vi "ResonanceAnalyzer.vi"() -> ()   [LabVIEW 2015]
uses:
  <vilib>/imath/engines/lvmath2/RunTimeEngine/Managers/WorkSpace/UID Generator.vi
  <vilib>/imath/engines/lvmath2/RunTimeEngine/RunTimeType/NIMS_RunTimeType_From StrictType (excl LVString).vi
  <instcachedir>/0/NIMS_RunTimeType_From StrictType (excl LVString)_EB1C38A9BC5048DA9ABDA8F781E54D21.lvgen/NIMS_RunTimeType_From StrictType (excl LVString)_EB1C38A9BC5048DA9ABDA8F781E54D21_000.vi
  <vilib>/imath/engines/lvmath2/RunTimeEngine/LocalVariableDefStatement/MC_LocalVariableDefStatement_Display.vi
  <vilib>/imath/engines/lvmath2/RunTimeEngine/Managers/SymbolTable/Clear UID.vi
  <vilib>/imath/engines/lvmath2/RunTimeEngine/NodeEndStatement/NIMS_NodeEndStatement_Output.vi
  <instcachedir>/0/NIMS_NodeEndStatement_Output_53EC0D466D134D7ABD903AC30B43404B.lvgen/NIMS_NodeEndStatement_Output_53EC0D466D134D7ABD903AC30B43404B_001.vi
  <vilib>/imath/engines/lvmath2/RunTimeEngine/ErrorHandling/NIMS_Finalize Error.vi
  <vilib>/Utility/file.llb/Read Delimited Spreadsheet (DBL).vi
  <vilib>/imath/engines/lvmath2/RunTimeEngine/Managers/SymbolTable/NIMS_WorkSpace.lvlib
panel:
  out "Array":dbl[](array[numeric])
  out "XY Graph":cluster{"all rows":dbl[], "all rows":dbl[]}(graph)
  in  "Tab Control":enum32{"Simulation", "Experiment"}(tab)
  in  "Input Parameters":T1
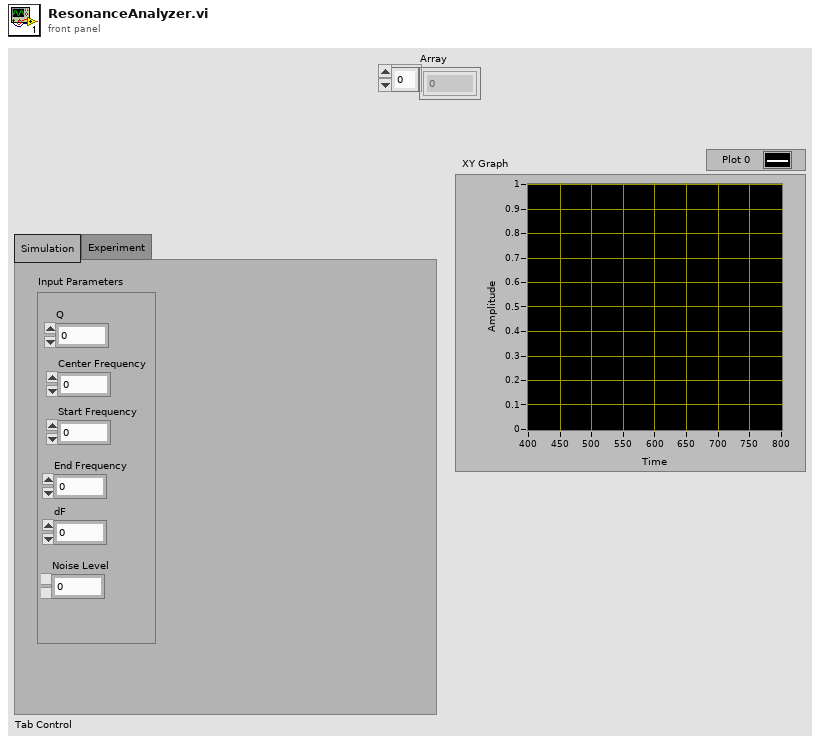
[diagram p1: front panel]
types:
  T1 = cluster{"Q":dbl, "Center Frequency":dbl, "Start Frequency":dbl, "End Frequency":dbl, "dF":dbl, "Noise Level":dbl}
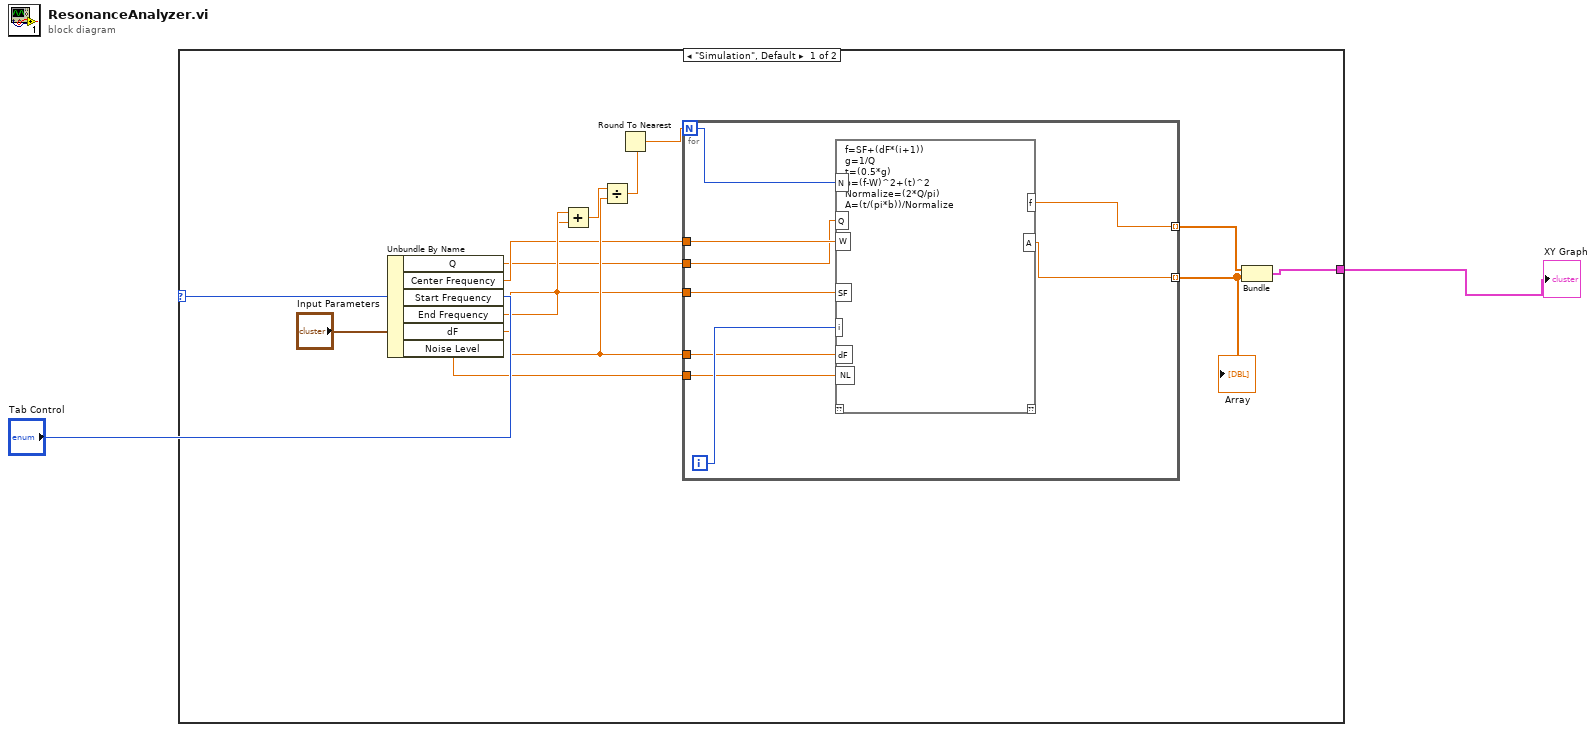
[diagram p0: block diagram]
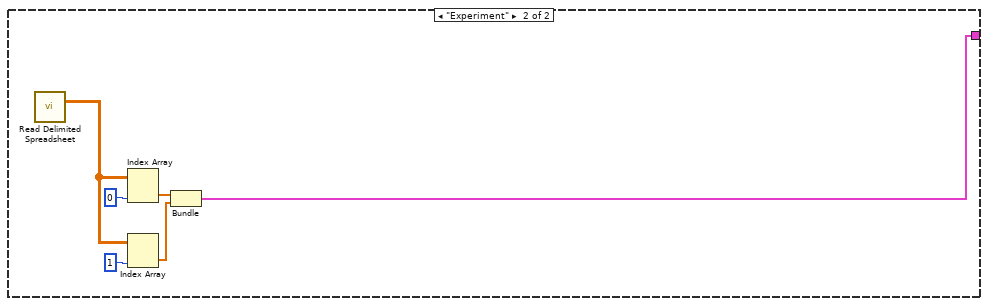
[diagram p2: hidden frame]
diagram:
  n1 = case shown="\"Simulation\", Default" "Tab Control" {
    tunnel: [w9 w164] -> w1
    frame "Simulation", Default {
      n2 = Unbundle By Name("Input Parameters") -> ("Q"=w4:dbl, "Center Frequency"=w5:dbl, "Start Frequency"=w6:dbl, "End Frequency"=w13:dbl, "dF"=w8:dbl, "Noise Level"=w7:dbl)
      n3 = Add(x=w13, y=w6) -> (x+y=w14:dbl)
      n4 = Divide(x=w14, y=w8) -> (x/y=w15:dbl)
      n5 = Round To Nearest(number=w15) -> (nearest integer value=w11:dbl)
      n6 = for {
        N: w11 -> [w18]
        tunnel: [w24] -> w10 mode=indexing
        tunnel: w8 -> [w22]
        tunnel: w7 -> [w21]
        tunnel: w6 -> [w20]
        tunnel: w5 -> [w19]
        tunnel: w4 -> [w17]
        tunnel: [w16] -> w3 mode=indexing
        i -> [w23]
        n7 = mathscript code="f=SF+(dF*(i+1))\ng=1/Q\nt=(0.5*g)\nb=(f-W)^2+(t)^2\nNormalize=(2*Q/pi)\nA=(t/(pi*b))/Normalize"("NL"=w21, "Q"=w17, "W"=w19, "N"=w18, "i"=w23, "SF"=w20, "dF"=w22) -> ("A"=w16:dbl, "f"=w24:dbl)  [unwired: 1 in, 1 out]
      }
      "Array" <- w3
      n8 = Bundle(w10, w3) -> (w9:cluster{dbl[], dbl[]})  [unwired: 1 in]
    }
    frame "Experiment" {
      n9 = call-poly <vilib>:"Read Delimited Spreadsheet.vi"() -> ("all rows"=w169:dbl[][])  [unwired: 10 in, 5 out]
      n10 = Index Array(array=w169, index (col)=0 ("disabled index (col)")) -> (element=w166:dbl[])  [unwired: 1 in]
      n11 = Index Array(array=w169, index (col)=1 ("disabled index (col)")) -> (element=w165:dbl[])  [unwired: 1 in]
      n12 = Bundle("all rows"=w166, "all rows"=w165) -> (w164:cluster{"all rows":dbl[], "all rows":dbl[]})  [unwired: 1 in]
    }
  }
  "XY Graph" <- w1
